vi "Falling Edge Detect (SubVI).vi"(11 "Input":bool=TRUE) -> (3 "Falling Edge?":bool)   [LabVIEW 2015]
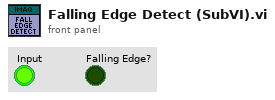
[diagram p1: front panel]
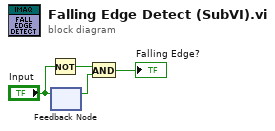
[diagram p0: block diagram]
diagram:
  n1 = Not(x="Input") -> (.not. x?=w2:bool)
  n2 = feedback #1() -> (w1:bool)  [unwired: 1 in]
  n3 = feedback-in #1("Input") -> ()
  n4 = And(x=w2, y=w1) -> (x .and. y?=→"Falling Edge?":bool)
